vi "Update Plot Legend.vi"(6 "Control Ref Queue":T1, 8 "error in (no error)":errorcluster, 10 "Multiplot Representation In":T2, 11 "2D Plot in":refnum<class "2D Plot.lvclass">) -> (0 "error out":errorcluster, 2 "Multiplot Representation Out":T2, 3 "2D Plot out":refnum<class "2D Plot.lvclass">)   [LabVIEW 2020, in "2D Plot.lvclass"]
uses:
  <vilib>/Math Plots/2D Math Plots/2D Plot/2D Plot/2D Plot.lvclass
  <vilib>/Math Plots/2D Math Plots/2D Plot/2D Plot/Typedef/Multiplot Representation.ctl
  <vilib>/Math Plots/2D Math Plots/2D Plot/2D Plot/Typedef/Plot Representation.ctl
  <vilib>/Math Plots/2D Math Plots/2D Plot/2D Plot/Typedef/Range Cluster.ctl
  <vilib>/Math Plots/2D Math Plots/2D Plot/Action String/2DMathPlot Ctrl Act Queue.ctl
  <vilib>/Math Plots/2D Math Plots/2D Plot/Action String/2DMathPlot Ctrl Act Cluster.ctl
  <vilib>/Math Plots/2D Math Plots/2D Plot/Action String/2DMathPlot State Class.ctl
  <vilib>/Math Plots/2D Math Plots/2D Plot/2D Plot/2D Plot.lvclass/2D Plot.ctl
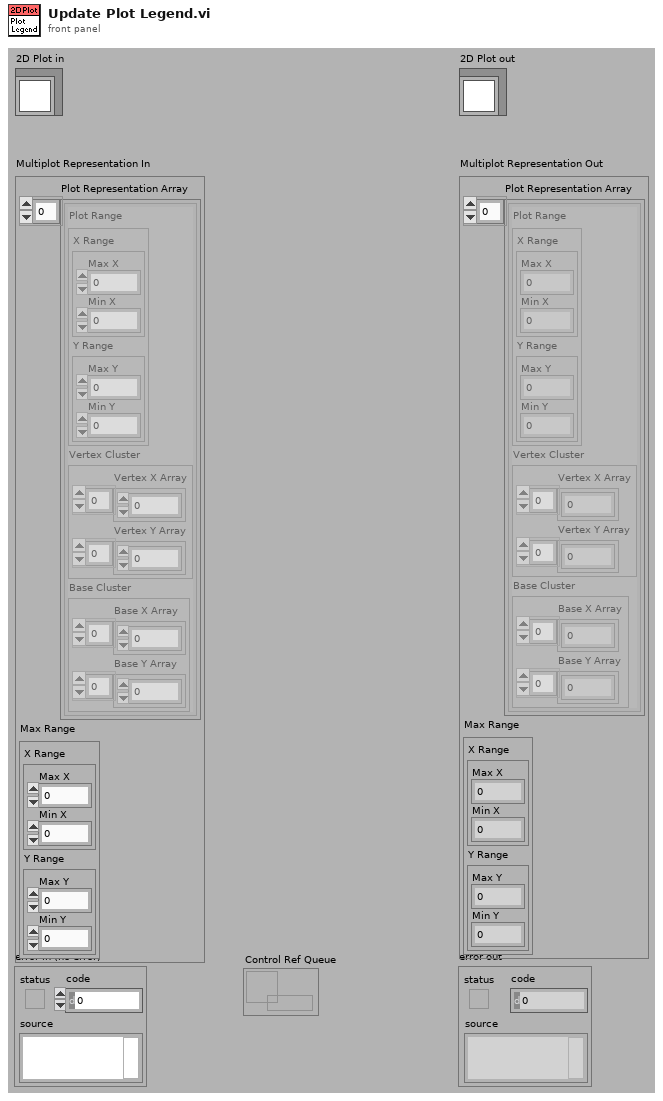
[diagram p1: front panel]
types:
  T1 = typedef "2DMathPlot Ctrl Act Queue.ctl" = refnum<queue>
  T2 = typedef "2D Plot.lvclass/Multiplot Representation.ctl" = cluster{"Plot Representation Array":T3[], "Max Range":T4}
  T3 = typedef "2D Plot.lvclass/Plot Representation.ctl" = cluster{"Plot Range":T4, "Vertex Cluster":cluster{"Vertex X Array":dbl[], "Vertex Y Array":dbl[]}, "Base Cluster":cluster{"Base X Array":dbl[], "Base Y Array":dbl[]}}
  T4 = typedef "2D Plot.lvclass/Range Cluster.ctl" = cluster{"X Range":cluster{"Max X":dbl, "Min X":dbl}, "Y Range":cluster{"Max Y":dbl, "Min Y":dbl}}
  T5 = typedef "2DMathPlot Ctrl Act Cluster.ctl" = cluster{"Plot Area Ref":refnum<vi>, "Z Axis Ref":refnum<vi>, "Legend Ref":refnum<vi>, "XControl Ref":refnum<vi>, "Facade Ref":refnum<vi>, "Display State Change Class":T6}
  T6 = typedef "2DMathPlot State Class.ctl" = enum16{"Update All (Undo)", "Update General", "Update Appearance", "Update Format", "Update Scale", "Update Marker", "Update Cursor", "None"}
  T7 = cluster{"Plot Name":string, "new picture":picture}[]
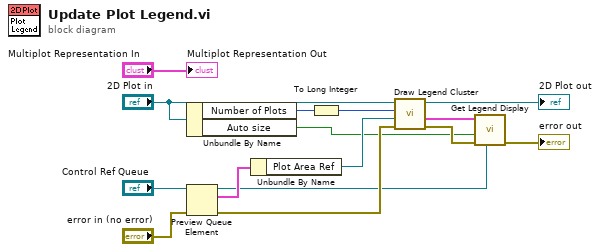
[diagram p0: block diagram]
diagram:
  n1 = Unbundle By Name("2D Plot in") -> ("Number of Plots"=w14:u32, "Auto size"=w1:bool)
  n2 = Preview Queue Element(queue="Control Ref Queue", error in (no error)="error in (no error)") -> (queue out=w5:T1, element=w15:T5, error out=w8:errorcluster)  [unwired: 2 out]
  n3 = Unbundle By Name(w15) -> ("Plot Area Ref"=w7:refnum<vi>)
  n4 = To Long Integer(number=w14) -> (32bit integer=w2:i32)
  n5 = call-dynamic "Draw Legend Cluster.vi"("error in (no error)"=w8, "Plot Area Ref"=w7, "Number Of Rows"=w2, "2D Plot in"="2D Plot in") -> ("error out"=w4:errorcluster, "Legend Cluster"=w6:T7, "2D Plot out"=→"2D Plot out":refnum<class "2D Plot.lvclass">)  [unwired: 1 in, 4 out]
  n6 = call <vilib>:"Get Legend Display.vi"("Control Ref Queue"=w5, "error in (no error)"=w4, "Auto Size?"=w1, "Legend Cluster"=w6) -> ("error out"=→"error out":errorcluster)  [unwired: 1 in, 6 out]
  "Multiplot Representation Out" <- "Multiplot Representation In"
